vi "fgv_Exp Stats.vi"(6 "Number of acquired frames":dbl, 7 "Ops":T2, 8 "error in (no error)":errorcluster, 9 "Acquisition time (ms)":dbl, 10 "Number of acquired data-points":dbl, 11 "Z-stack duration (sec)":dbl) -> (0 "error out":errorcluster, 3 "STATISTICS":T1)   [LabVIEW 2020]
uses:
  User Interface/Visualisation/Functional Imaging Viewer/SubVIs/Experiment header interface/Typedefs/Header subclusters/Header params-statistics.ctl
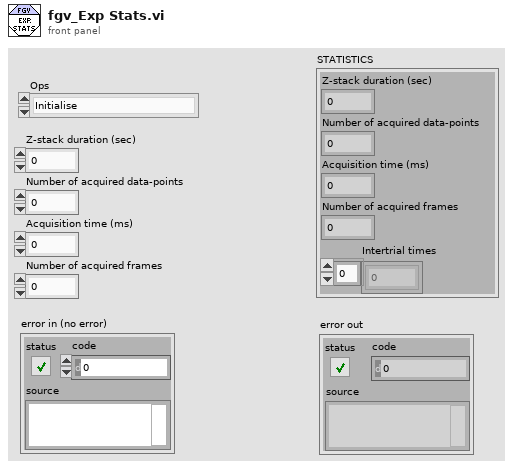
[diagram p1: front panel]
types:
  T1 = typedef "Header params-statistics.ctl" = cluster{"Z-stack duration (sec)":dbl, "Number of acquired data-points":dbl, "Acquisition time (ms)":dbl, "Number of acquired frames":dbl, "Intertrial times":dbl[]}
  T2 = typedef "fgv_Exp Stats ops" = enum16{"Initialise", "Update Z-stack duration", "Update no. of acqd pts", "Update Acq time", "Update no of acqd frames", "Read", "Clear"}
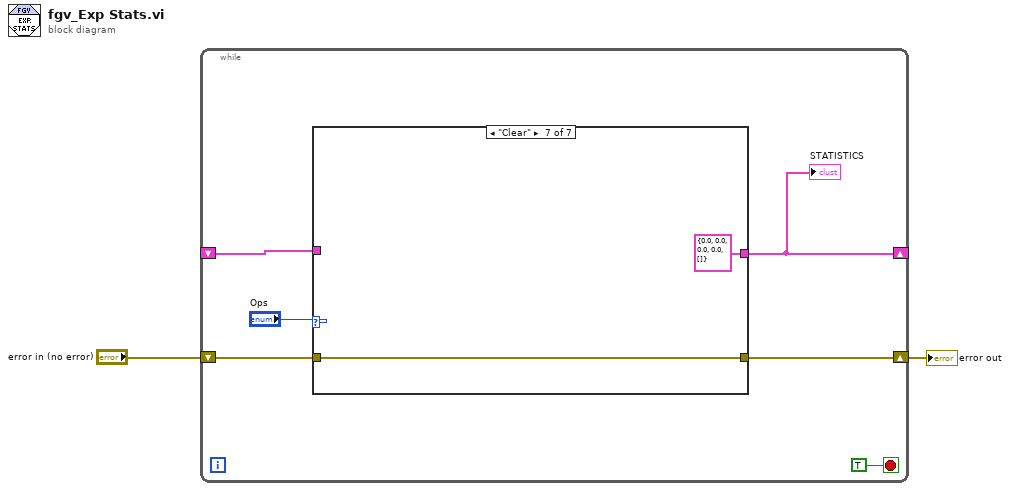
[diagram p0: block diagram]
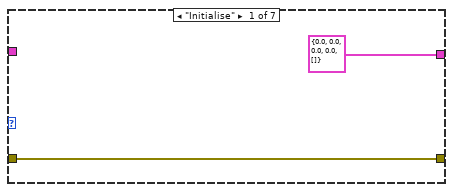
[diagram p2: hidden frame]
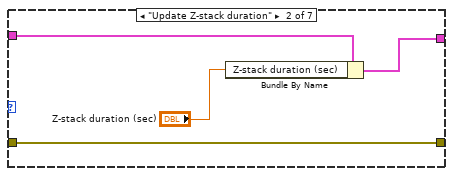
[diagram p3: hidden frame]
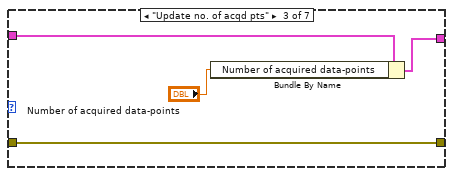
[diagram p4: hidden frame]
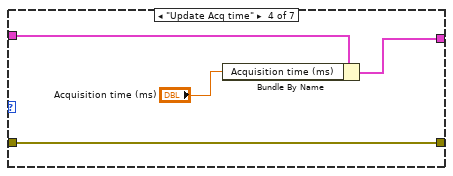
[diagram p5: hidden frame]
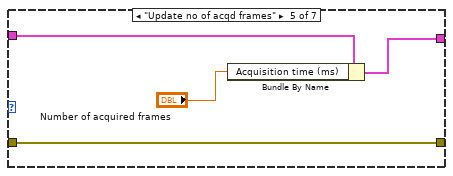
[diagram p6: hidden frame]
diagram:
  n1 = while {
    shift-right: [w7] -> _
    shift-left: _ -> [w6]
    shift-right: [w4] -> w1
    shift-left: "error in (no error)" -> [w5]
    stop <- TRUE stop-if-true
    n2 = case shown="\"Clear\"" "Ops" {
      tunnel: [T1 {"Z-stack duration (sec)"=0.0, "Number of acquired data-points"=0.0, "Acquisition time (ms)"=0.0, "Number of acquired frames"=0.0, "Intertrial times"=[]} ("STATISTICS 2") w13 w17 w21 w25 w27 T1 {"Z-stack duration (sec)"=0.0, "Number of acquired data-points"=0.0, "Acquisition time (ms)"=0.0, "Number of acquired frames"=0.0, "Intertrial times"=[]} ("STATISTICS 2")] -> w7
      tunnel: w6 -> [_ w14 w18 w22 w26 w27 _]
      tunnel: [w9 w12 w15 w19 w23 w28 w30] -> w4
      tunnel: w5 -> [w9 w12 w15 w19 w23 w28 w30]
      frame "Initialise" {
      }
      frame "Update Z-stack duration" {
        n3 = Bundle By Name(cluster=w14, "Z-stack duration (sec)"="Z-stack duration (sec)") -> (w13:T1)
      }
      frame "Update no. of acqd pts" {
        n4 = Bundle By Name(cluster=w18, "Number of acquired data-points"="Number of acquired data-points") -> (w17:T1)
      }
      frame "Update Acq time" {
        n5 = Bundle By Name(cluster=w22, "Acquisition time (ms)"="Acquisition time (ms)") -> (w21:T1)
      }
      frame "Update no of acqd frames" {
        n6 = Bundle By Name(cluster=w26, "Acquisition time (ms)"="Number of acquired frames") -> (w25:T1)
      }
      frame "Read", Default {
      }
      frame "Clear" {
      }
    }
    "STATISTICS" <- w7
  }
  "error out" <- w1
